vi "DHE_CheckCommandTmout.vi"(5 "arguments":string, 6 "phys. unit":string, 7 "DBSRef":T1, 9 "Command":string, 10 "TimeOut in":i32=30000) -> (1 "TimeOut out":i32=30000, 3 "command out":string)   [LabVIEW 2016]
uses:
  DBSHAND/private/vis/DatabaseHand_RefNum.ctl
  DBSHAND/private/vis/DatabaseHand_Element_Get(bool).vi
panel:
  out "sur":i32
  out "nimages":i32=1
  out "fsamples":i32=1
  out "coadds":i32=1
  out "exposuretime":i32
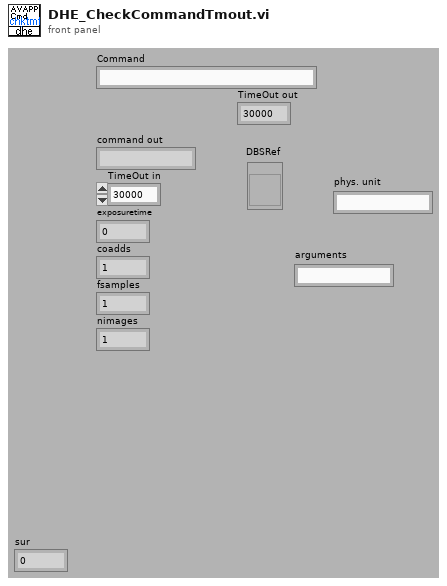
[diagram p1: front panel]
types:
  T1 = typedef "DatabaseHand_RefNum.ctl" = refnum<vi>
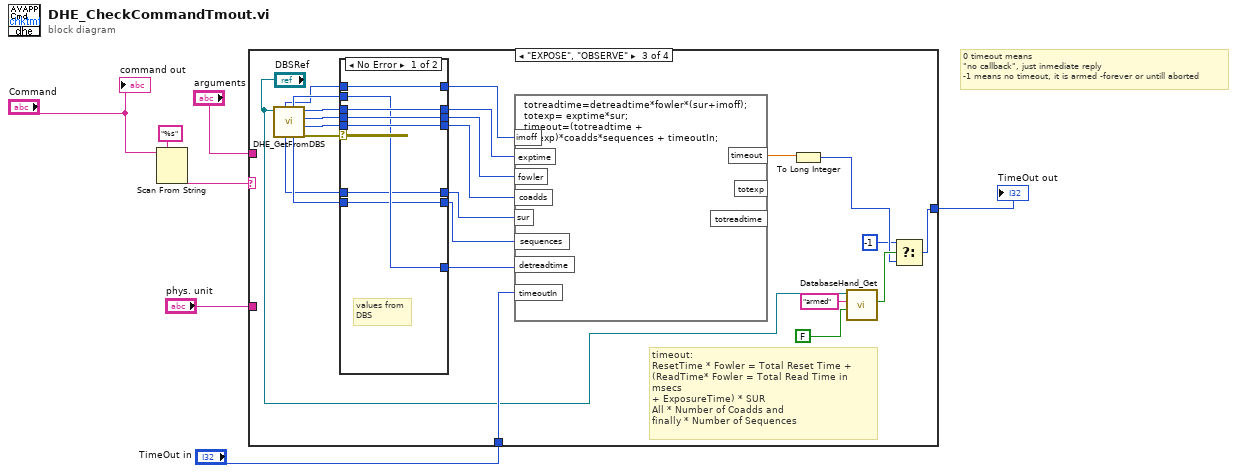
[diagram p0: block diagram]
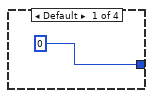
[diagram p2: hidden frame]
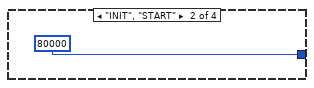
[diagram p3: hidden frame]
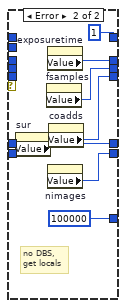
[diagram p4: hidden frame]
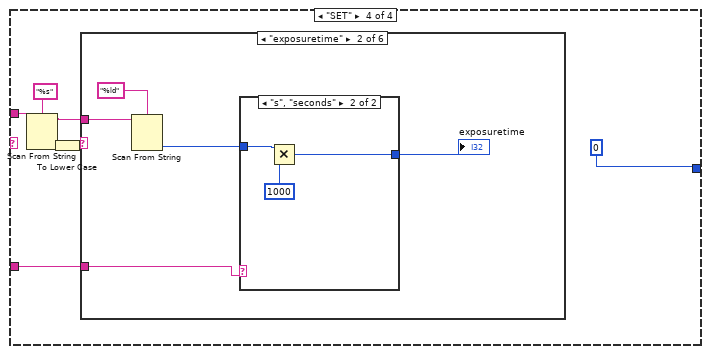
[diagram p5: hidden frame]
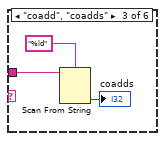
[diagram p8: hidden frame]
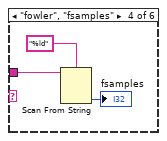
[diagram p9: hidden frame]
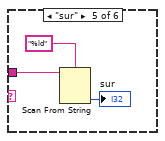
[diagram p10: hidden frame]
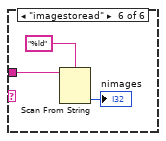
[diagram p11: hidden frame]
diagram:
  # "0 timeout means\n\"no callback\", just inmediate reply\n-1 means no timeout, it is armed -forever or untill aborted"
  n1 = Scan From String(format string="%s" ("Format String"), input string="Command") -> (output 1=w4:string)  [unwired: 2 in, 4 out]
  n2 = case shown="\"EXPOSE\", \"OBSERVE\"" w4 {
    tunnel: "TimeOut in" -> [_ _ w19 _]
    tunnel: "arguments" -> [_ _ _ w54]
    tunnel: "phys. unit" -> [_ _ _ w50]
    tunnel: [u32 0 ("TimeOut in") u32 80000 ("TimeOut in") w12 u32 0 ("TimeOut in")] -> w1
    frame Default {
    }
    frame "INIT", "START" {
    }
    frame "EXPOSE", "OBSERVE" {
      # "timeout:\nResetTime * Fowler = Total Reset Time +\n(ReadTime* Fowler = Total Read Time in msecs\n+ ExposureTime) * SUR \nAll * Number of Coadds and\nfinally * Number of Sequences"
      n3 = call "DHE_GetFromDBS.vi"("Database RefNum in"="DBSRef") -> ("error out"=w33:errorcluster, "coadds"=w30:i32, "fsamples"=w31:i32, "exptime"=w32:i32, "nimages"=w28:i32, "readtime"=w29:i32, "sur"=w27:i32, "image_factor"=w11:i32)  [unwired: 1 in, 2 out]
      n4 = case shown="No Error" w33 {
        tunnel: [w40 w47] -> w26
        tunnel: w32 -> [w40 _]
        tunnel: [w39 w46] -> w25
        tunnel: w31 -> [w39 _]
        tunnel: [w38 w45] -> w24
        tunnel: w30 -> [w38 _]
        tunnel: w29 -> [w37 _]
        tunnel: [w37 100000 ("readtime")] -> w21
        tunnel: [w36 w43] -> w22
        tunnel: w28 -> [w36 _]
        tunnel: w27 -> [w35 _]
        tunnel: [w35 w42] -> w23
        tunnel: w11 -> [w34 _]
        tunnel: [w34 1 ("factor")] -> w10
        frame No Error {
          # "values from\nDBS"
        }
        frame Error {
          # "no DBS,\nget locals"
          n5 = property on="sur" class="DigNum (strict)"() -> ("Value"=w42:i32)  [unwired: 2 in, 2 out]
          n6 = property on="fsamples" class="DigNum (strict)"() -> ("Value"=w46:i32)  [unwired: 2 in, 2 out]
          n7 = property on="exposuretime" class="DigNum (strict)"() -> ("Value"=w47:i32)  [unwired: 2 in, 2 out]
          n8 = property on="nimages" class="DigNum (strict)"() -> ("Value"=w43:i32)  [unwired: 2 in, 2 out]
          n9 = property on="coadds" class="DigNum (strict)"() -> ("Value"=w45:i32)  [unwired: 2 in, 2 out]
        }
      }
      n10 = formula code="totreadtime=detreadtime*fowler*(sur+imoff);\ntotexp= exptime*sur;\ntimeout=(totreadtime + totexp)*coadds*sequences + timeoutIn;"("exptime"=w26, "fowler"=w25, "coadds"=w24, "sur"=w23, "sequences"=w22, "detreadtime"=w21, "timeoutIn"=w19, "imoff"=w10) -> ("timeout"=w20:dbl)  [unwired: 2 out]
      n11 = To Long Integer(number=w20) -> (32bit integer=w14:i32)
      n12 = call-poly "DatabaseHand_Get.vi"("default value"=FALSE, "name"="armed", "Database RefNum in"="DBSRef") -> ("value"=w15:bool)  [unwired: 2 in, 6 out]
      n13 = Select(t=-1, s=w15, f=w14) -> (s? t:f=w12:i32)
    }
    frame "SET" {
      n14 = Scan From String(format string="%s", input string=w54) -> (remaining string=w49:string, output 1=w53:string)  [unwired: 2 in, 3 out]
      n15 = To Lower Case(string=w53) -> (all lower case string=w51:string)
      n16 = case shown="\"exposuretime\"" w51 {
        tunnel: w49 -> [_ w59 w66 w69 w72 w75]
        tunnel: w50 -> [_ w57 _ _ _ _]
        frame Default {
        }
        frame "exposuretime" {
          n17 = Scan From String(format string="%ld", input string=w59) -> (output 1=w56:i32)  [unwired: 2 in, 4 out]
          n18 = case shown="\"s\", \"seconds\"" w57 {
            tunnel: w56 -> [w60 w63]
            tunnel: [w60 w61] -> w55
            frame Default {
            }
            frame "s", "seconds" {
              n19 = Multiply(x=w63, y=1000) -> (x*y=w61:i32)
            }
          }
          "exposuretime" <- w55
        }
        frame "coadd", "coadds" {
          n20 = Scan From String(format string="%ld", input string=w66) -> (output 1=→"coadds":i32)  [unwired: 2 in, 4 out]
        }
        frame "fowler", "fsamples" {
          n21 = Scan From String(format string="%ld", input string=w69) -> (output 1=→"fsamples":i32)  [unwired: 2 in, 4 out]
        }
        frame "sur" {
          n22 = Scan From String(format string="%ld", input string=w72) -> (output 1=→"sur":i32)  [unwired: 2 in, 4 out]
        }
        frame "imagestoread" {
          n23 = Scan From String(format string="%ld", input string=w75) -> (output 1=→"nimages":i32)  [unwired: 2 in, 4 out]
        }
      }
    }
  }
  "TimeOut out" <- w1
  "command out" <- "Command"
